vi "observacao_0MQ.vi"() -> ()   [LabVIEW 2012, in "Shared_160.lvlib"] (continued)
                n1514 = Multiply(x=0.01745329252 ("y"), y=w1906) -> (x*y=w1905:dbl)
                n1515 = Cosine(x=w1905) -> (cos(x)=w1894:dbl)
                n1516 = Sine(x=w1905) -> (sin(x)=w1895:dbl)
                n1517 = Multiply(x=w1892, y=w1894) -> (x*y=w1886:dbl)
                n1518 = Multiply(x=w1894, y=w1893) -> (x*y=w1891:dbl)
                n1519 = Multiply(x=w1893, y=w1895) -> (x*y=w1887:dbl)
                n1520 = Multiply(x=w1895, y=w1892) -> (x*y=w1890:dbl)
                n1521 = Subtract(x=w1891, y=w1890) -> (x-y=w1889:dbl)
                n1522 = Add(x=w1887, y=w1886) -> (x+y=w1888:dbl)
                n1523 = Less Than 0?(x=w1889) -> (x < 0?=w1903:bool)
                n1524 = Less Than 0?(x=w1888) -> (x < 0?=w1899:bool)
                n1525 = case shown="True" w1899 {
                  tunnel: w1897 -> [w1923 w1926]
                  tunnel: [w1922 w1927] -> w1896
                  frame False {
                    n1526 = Select(t="W" ("y"), s=w1923, f="E" ("y")) -> (s? t:f=w1922:string)
                  }
                  frame True {
                    n1527 = Select(t="E" ("y"), s=w1926, f="W" ("y")) -> (s? t:f=w1927:string)
                  }
                }
                n1528 = Select(t="S" ("y"), s=w1903, f="N" ("y")) -> (s? t:f=w1902:string)
                n1529 = Absolute Value(x=w1889) -> (abs(x)=w1900:dbl)
                n1530 = Absolute Value(x=w1888) -> (abs(x)=w1898:dbl)
                n1531 = global write "Global_Telescopio.vi" "guide_dir_we"(w1896) -> ()
                n1532 = global write "Global_Telescopio.vi" "guide_dir_ns"(w1902) -> ()
                n1533 = global write "Global_Telescopio.vi" "guide_dec"(w1900) -> ()
                n1534 = global write "Global_Telescopio.vi" "guide_asc"(w1898) -> ()
              }
            }
            "LED VAR TRACKING" <- "VARIABLE \nTRACKING"
          }
          frame "CALIBRATION" {
            # "Alterado dia 23/07/218"
            n1535 = disable-structure shown="Disabled" {
              frame Disabled {
              }
              frame Enabled {
              }
            }
            n1536 = disable-structure shown="Disabled" {
              frame Disabled {
                w1960 = u16 4 items=["ZERO", "AH", "DEC", "TUBO", "CUP"] ("Controlador")
                n1537 = call "Monta Comando.vi"("Comando"="FECHAR", "Dispositivo"="TRAPEIRA" ("Comando"), "Controlador"=w1960) -> ()  [unwired: 4 in, 3 out]
              }
              frame Enabled {
              }
            }
            n1538 = event shown="[4] \"Coude\": Value Change" {
              selector: _ -> [_ _ _ _ _]
              dyn-events: _ -> [_ _ _ _ _]
              timeout: 10 -> [_ _ _ _ _]
              event Timeout {
                n1539 = event-data() -> ()  [unwired: 1 in, 2 out]
              }
              event "Weak": Value Change {
                w1963 = u16 6 items=["Alarme", "Atencao", "Erro", "Ocupado", "TBD", "LCB", "Trapeira", "Paravento", "DomoRap", "DomoCW", "DomoCCW", "TBD", "Em movimento", "TBD"] ("NomeStatus")
                n1540 = event-data() -> ("NewVal"=w1964:bool)  [unwired: 1 in, 5 out]
                n1541 = call "Bit Status CUP.vi"("NomeStatus"=w1963) -> ("StatBit"=w1962:bool)
                n1542 = case shown="False" w1962 {
                  tunnel: w1964 -> [w1971 _]
                  frame False {
                    w1965 = u16 4 items=["ZERO", "AH", "DEC", "TUBO", "CUP"] ("Controlador")
                    n1543 = case shown="True" w1971 {
                      tunnel: [w1972 TRUE ("WeakSel")] -> w1970
                      tunnel: [w1972 FALSE ("MediumSel")] -> w1968
                      tunnel: [0 2] -> w1967
                      tunnel: ["DESLIGAR" ("Comando") "LIGAR" ("Comando")] -> w1969
                      frame False {
                        w1972 = FALSE ("MediumSel")
                      }
                      frame True {
                        n1544 = local write "DOME"(FALSE) -> ()
                        n1545 = local write "StatShutter"("Busy to Close" ("Status")) -> ()
                      }
                    }
                    n1546 = property on="Coude" class="Bool (strict)"("DisabledEnum"=w1967) -> ()  [unwired: 2 in, 2 out]
                    n1547 = property on="WeakSel" class="Bool (strict)"("Value"=w1970) -> ()  [unwired: 2 in, 2 out]
                    n1548 = property on="CoudeSel" class="Bool (strict)"("Value"=w1968) -> ()  [unwired: 2 in, 2 out]
                    n1549 = property on="Strong" class="Bool (strict)"("Disabled"=w1967) -> ()  [unwired: 2 in, 2 out]
                    n1550 = property on="MediumSel" class="Bool (strict)"("Value"=w1968) -> ()  [unwired: 2 in, 2 out]
                    n1551 = property on="StrongSel" class="Bool (strict)"("Value"=w1968) -> ()  [unwired: 2 in, 2 out]
                    n1552 = property on="Medium" class="Bool (strict)"("Disabled"=w1967) -> ()  [unwired: 2 in, 2 out]
                    n1553 = call "Monta Comando.vi"("Comando"=w1969, "Dispositivo"="FLAT_WEAK", "Controlador"=w1965) -> ()  [unwired: 4 in, 3 out]
                  }
                  frame True {
                    w1981 = FALSE ("Weak")
                    n1554 = Get Date/Time In Seconds() -> (seconds since 1Jan1904=w1984:timestamp)
                    n1555 = Add(x=w1984, y=10.0) -> (x+y=w1985:timestamp)
                    n1556 = property on="Weak" class="Bool (strict)"("Value"=w1981) -> ()  [unwired: 2 in, 2 out]
                    n1557 = local write "alarm Time"(w1985) -> ()
                    n1558 = property on="Mensage Alarme" class="Str"("Visible"=TRUE) -> ()  [unwired: 2 in, 2 out]
                    n1559 = property on="WeakSel" class="Bool (strict)"("Value"=w1981) -> ()  [unwired: 2 in, 2 out]
                    n1560 = local write "Flag Alarm"(TRUE ("Flag Alarm")) -> ()
                  }
                }
              }
              event "Medium": Value Change {
                w1988 = u16 6 items=["Alarme", "Atencao", "Erro", "Ocupado", "TBD", "LCB", "Trapeira", "Paravento", "DomoRap", "DomoCW", "DomoCCW", "TBD", "Em movimento", "TBD"] ("NomeStatus")
                n1561 = event-data() -> ("NewVal"=w1989:bool)  [unwired: 1 in, 5 out]
                n1562 = call "Bit Status CUP.vi"("NomeStatus"=w1988) -> ("StatBit"=w1987:bool)
                n1563 = case shown="False" w1987 {
                  tunnel: w1989 -> [w1996 _]
                  frame False {
                    w1991 = u16 4 items=["ZERO", "AH", "DEC", "TUBO", "CUP"] ("Controlador")
                    n1564 = case shown="True" w1996 {
                      tunnel: [0 2] -> w1993
                      tunnel: [w1998 TRUE] -> w1994
                      tunnel: [w1998 FALSE] -> w1992
                      tunnel: ["DESLIGAR" "LIGAR"] -> w1995
                      frame False {
                        w1998 = FALSE
                      }
                      frame True {
                        n1565 = local write "DOME"(FALSE) -> ()
                        n1566 = local write "StatShutter"("Busy to Close" ("Status")) -> ()
                      }
                    }
                    n1567 = property on="Weak" class="Bool (strict)"("Disabled"=w1993) -> ()  [unwired: 2 in, 2 out]
                    n1568 = property on="Strong" class="Bool (strict)"("Disabled"=w1993) -> ()  [unwired: 2 in, 2 out]
                    n1569 = property on="WeakSel" class="Bool (strict)"("Value"=w1992) -> ()  [unwired: 2 in, 2 out]
                    n1570 = property on="MediumSel" class="Bool (strict)"("Value"=w1994) -> ()  [unwired: 2 in, 2 out]
                    n1571 = property on="StrongSel" class="Bool (strict)"("Value"=w1992) -> ()  [unwired: 2 in, 2 out]
                    n1572 = property on="Coude" class="Bool (strict)"("DisabledEnum"=w1993) -> ()  [unwired: 2 in, 2 out]
                    n1573 = property on="CoudeSel" class="Bool (strict)"("Value"=w1992) -> ()  [unwired: 2 in, 2 out]
                    n1574 = call "Monta Comando.vi"("Comando"=w1995, "Dispositivo"="FLAT_LO", "Controlador"=w1991) -> ()  [unwired: 4 in, 3 out]
                  }
                  frame True {
                    w2006 = FALSE ("Medium")
                    n1575 = Get Date/Time In Seconds() -> (seconds since 1Jan1904=w2009:timestamp)
                    n1576 = Add(x=w2009, y=10.0) -> (x+y=w2010:timestamp)
                    n1577 = local write "alarm Time"(w2010) -> ()
                    n1578 = property on="Mensage Alarme" class="Str"("Visible"=TRUE) -> ()  [unwired: 2 in, 2 out]
                    n1579 = local write "Flag Alarm"(TRUE ("Flag Alarm")) -> ()
                    n1580 = property on="Medium" class="Bool (strict)"("Value"=w2006) -> ()  [unwired: 2 in, 2 out]
                    n1581 = property on="MediumSel" class="Bool (strict)"("Value"=w2006) -> ()  [unwired: 2 in, 2 out]
                  }
                }
              }
              event "Strong": Value Change {
                w2013 = u16 6 items=["Alarme", "Atencao", "Erro", "Ocupado", "TBD", "LCB", "Trapeira", "Paravento", "DomoRap", "DomoCW", "DomoCCW", "TBD", "Em movimento", "TBD"] ("NomeStatus")
                n1582 = event-data() -> ("NewVal"=w2014:bool)  [unwired: 1 in, 5 out]
                n1583 = call "Bit Status CUP.vi"("NomeStatus"=w2013) -> ("StatBit"=w2012:bool)
                n1584 = case shown="False" w2012 {
                  tunnel: w2014 -> [w2022 _]
                  frame False {
                    w2015 = u16 4 items=["ZERO", "AH", "DEC", "TUBO", "CUP"] ("Controlador")
                    n1585 = case shown="True" w2022 {
                      tunnel: [FALSE w2030] -> w2017
                      tunnel: [w2023 w2030] -> w2021
                      tunnel: [0 2] -> w2018
                      tunnel: ["DESLIGAR" "LIGAR"] -> w2020
                      tunnel: [w2023 TRUE] -> w2019
                      frame False {
                        w2023 = FALSE
                      }
                      frame True {
                        w2030 = FALSE
                        n1586 = local write "DOME"(FALSE) -> ()
                        n1587 = local write "StatShutter"("Busy to Close" ("Status")) -> ()
                      }
                    }
                    n1588 = property on="Medium" class="Bool (strict)"("Disabled"=w2018) -> ()  [unwired: 2 in, 2 out]
                    n1589 = property on="Weak" class="Bool (strict)"("Disabled"=w2018) -> ()  [unwired: 2 in, 2 out]
                    n1590 = property on="WeakSel" class="Bool (strict)"("Value"=w2021) -> ()  [unwired: 2 in, 2 out]
                    n1591 = property on="MediumSel" class="Bool (strict)"("Value"=w2017) -> ()  [unwired: 2 in, 2 out]
                    n1592 = property on="StrongSel" class="Bool (strict)"("Value"=w2019) -> ()  [unwired: 2 in, 2 out]
                    n1593 = property on="Coude" class="Bool (strict)"("DisabledEnum"=w2018) -> ()  [unwired: 2 in, 2 out]
                    n1594 = property on="CoudeSel" class="Bool (strict)"("Value"=w2017) -> ()  [unwired: 2 in, 2 out]
                    n1595 = call "Monta Comando.vi"("Comando"=w2020, "Dispositivo"="FLAT_HI", "Controlador"=w2015) -> ()  [unwired: 4 in, 3 out]
                  }
                  frame True {
                    w2033 = FALSE ("Strong")
                    n1596 = property on="StrongSel" class="Bool (strict)"("Value"=w2033) -> ()  [unwired: 2 in, 2 out]
                    n1597 = property on="Strong" class="Bool (strict)"("Value"=w2033) -> ()  [unwired: 2 in, 2 out]
                    n1598 = Get Date/Time In Seconds() -> (seconds since 1Jan1904=w2036:timestamp)
                    n1599 = Add(x=w2036, y=10.0) -> (x+y=w2037:timestamp)
                    n1600 = local write "alarm Time"(w2037) -> ()
                    n1601 = property on="Mensage Alarme" class="Str"("Visible"=TRUE) -> ()  [unwired: 2 in, 2 out]
                    n1602 = local write "Flag Alarm"(TRUE ("Flag Alarm")) -> ()
                  }
                }
              }
              event "Coude": Value Change {
                w2040 = u16 6 items=["Alarme", "Atencao", "Erro", "Ocupado", "TBD", "LCB", "Trapeira", "Paravento", "DomoRap", "DomoCW", "DomoCCW", "TBD", "Em movimento", "TBD"] ("NomeStatus")
                n1603 = event-data() -> ("NewVal"=w2041:bool)  [unwired: 1 in, 5 out]
                n1604 = call "Bit Status CUP.vi"("NomeStatus"=w2040) -> ("StatBit"=w2039:bool)
                n1605 = case shown="False" w2039 {
                  tunnel: w2041 -> [w2048 _]
                  frame False {
                    w2042 = u16 4 items=["ZERO", "AH", "DEC", "TUBO", "CUP"] ("Controlador")
                    n1606 = case shown="True" w2048 {
                      tunnel: [FALSE w2057] -> w2045
                      tunnel: [w2050 w2057] -> w2046
                      tunnel: [0 2] -> w2044
                      tunnel: ["DESLIGAR" "LIGAR"] -> w2049
                      tunnel: [w2050 TRUE] -> w2047
                      frame False {
                        w2050 = FALSE
                      }
                      frame True {
                        w2057 = FALSE
                        n1607 = local write "DOME"(FALSE) -> ()
                        n1608 = local write "StatShutter"("Busy to Close" ("Status")) -> ()
                      }
                    }
                    n1609 = property on="StrongSel" class="Bool (strict)"("Value"=w2046) -> ()  [unwired: 2 in, 2 out]
                    n1610 = property on="CoudeSel" class="Bool (strict)"("Value"=w2047) -> ()  [unwired: 2 in, 2 out]
                    n1611 = property on="MediumSel" class="Bool (strict)"("Value"=w2045) -> ()  [unwired: 2 in, 2 out]
                    n1612 = property on="Weak" class="Bool (strict)"("DisabledEnum"=w2044) -> ()  [unwired: 2 in, 2 out]
                    n1613 = property on="Medium" class="Bool (strict)"("DisabledEnum"=w2044) -> ()  [unwired: 2 in, 2 out]
                    n1614 = property on="Strong" class="Bool (strict)"("DisabledEnum"=w2044) -> ()  [unwired: 2 in, 2 out]
                    n1615 = property on="WeakSel" class="Bool (strict)"("Value"=w2045) -> ()  [unwired: 2 in, 2 out]
                    n1616 = call "Monta Comando.vi"("Comando"=w2049, "Dispositivo"="FLAT_COUDE", "Controlador"=w2042) -> ()  [unwired: 4 in, 3 out]
                  }
                  frame True {
                    w2060 = FALSE ("Coude")
                    n1617 = Get Date/Time In Seconds() -> (seconds since 1Jan1904=w2063:timestamp)
                    n1618 = Add(x=w2063, y=10.0) -> (x+y=w2064:timestamp)
                    n1619 = local write "alarm Time"(w2064) -> ()
                    n1620 = property on="Mensage Alarme" class="Str"("Visible"=TRUE) -> ()  [unwired: 2 in, 2 out]
                    n1621 = local write "Flag Alarm"(TRUE ("Flag Alarm")) -> ()
                    n1622 = property on="CoudeSel" class="Bool (strict)"("Value"=w2060) -> ()  [unwired: 2 in, 2 out]
                    n1623 = property on="Coude" class="Bool (strict)"("Value"=w2060) -> ()  [unwired: 2 in, 2 out]
                  }
                }
              }
            }
          }
          frame "LIST" {
            n1624 = stacked-sequence {
              frame #0 {
                # "Muda nome do controle de RA para AH se MAFmax == 100"
                n1625 = case shown="True" "SET coord" {
                  frame False {
                  }
                  frame True {
                    n1626 = stacked-sequence {
                      frame #0 {
                        w2081 = "2000"
                        # "Valores aux para Detectar Edição"
                        n1627 = local read "Multicolumn Listbox"() -> (w2088:i32[])
                        n1628 = property on="Multicolumn Listbox" class="MCListbox (strict)"() -> ("Item Names"=w2086:string[][])  [unwired: 2 in, 2 out]
                        n1629 = Index Array(array=w2088, index=0) -> (element=w2085:i32)
                        n1630 = local write "FLAG SET COORD"(TRUE ("FLAG_MAG")) -> ()
                        n1631 = Index Array(array=w2086, index (row)=w2085) -> (element=w2084:string[])  [unwired: 1 in]
                        n1632 = Index Array(array=w2084, index #1=0 ("index")) -> (element #1=w2077:string, element #2=w2075:string, element #3=w2076:string, element #4=w2078:string, element #5=w2080:string, element #6=w2079:string)  [unwired: 5 in]
                        "RA AUX" <- w2075
                        "AUX EDITA Name" <- w2077
                        "AUX EDITA RA" <- w2075
                        "AUX EDITA DEC" <- w2076
                        "AUX EDITA PMRA" <- w2080
                        "AUX EDITA PMDEC" <- w2079
                        n1633 = local write "StrPointObjPMRA"(w2080) -> ()
                        n1634 = local write "StrPointObjPMDEC"(w2079) -> ()
                        n1635 = local write "StrPointObjName"(w2077) -> ()
                        n1636 = local write "StrPointObjRA"(w2075) -> ()
                        n1637 = local write "StrPointObjDEC"(w2076) -> ()
                        n1638 = local write "MAG"(w2078) -> ()
                        n1639 = local write "StrPointObjEpoch"(w2081) -> ()
                        "EPOCH AUX" <- w2081
                        "AUX EDITA EPOCH" <- w2081
                      }
                      frame #1 {
                        n1640 = case shown="False" "Case Constant\n(See Context Help) 7" {
                          frame False {
                          }
                          frame True {
                            # "Ao clicar SET COORD, fechar a aba LIST e abrir a aba POINTING"
                            n1641 = local write "Setup, Pointing & Guiding"(T2."POINTING" ("Setup, Pointing & Guiding")) -> ()
                          }
                        }
                      }
                    }
                  }
                }
                n1642 = case shown="True" "Clear ALL" {
                  frame False {
                  }
                  frame True {
                    n1643 = Two Button Dialog(message="Will you clear All Table?") -> (T button?=w2091:bool)  [unwired: 2 in]
                    n1644 = case shown="True" w2091 {
                      frame False {
                      }
                      frame True {
                        w2093 = string[][] [] ("Item Names")
                        # "Limpa a Tabela Inteira"
                        n1645 = property on="Multicolumn Listbox" class="MCListbox (strict)"("Item Names"=w2093) -> ()  [unwired: 2 in, 2 out]
                        n1646 = local write "subarray"(w2093) -> ()
                      }
                    }
                  }
                }
                n1647 = local read "MAG Max"() -> (w2067:dbl)
                n1648 = Equal?(x=100.0, y=w2067) -> (x = y?=w2066:bool)
                n1649 = case shown="False" w2066 {
                  frame False {
                    n1650 = flat-sequence {
                      frame #0 {
                        w2071 = FALSE
                        n1651 = property on="RA Max" class="DigNum (strict)"("Caption.Visible"=w2071) -> ()  [unwired: 2 in, 2 out]
                        n1652 = property on="RA Min" class="DigNum (strict)"("Caption.Visible"=w2071) -> ()  [unwired: 2 in, 2 out]
                      }
                      frame #1 {
                        w2072 = TRUE
                        n1653 = property on="RA Min" class="DigNum (strict)"("Label.Visible"=w2072) -> ()  [unwired: 2 in, 2 out]
                        n1654 = property on="RA Max" class="DigNum (strict)"("Label.Visible"=w2072) -> ()  [unwired: 2 in, 2 out]
                      }
                    }
                  }
                  frame True {
                    n1655 = flat-sequence {
                      frame #0 {
                        w2073 = FALSE
                        n1656 = property on="RA Max" class="DigNum (strict)"("Label.Visible"=w2073) -> ()  [unwired: 2 in, 2 out]
                        n1657 = property on="RA Min" class="DigNum (strict)"("Label.Visible"=w2073) -> ()  [unwired: 2 in, 2 out]
                      }
                      frame #1 {
                        w2074 = TRUE
                        n1658 = property on="RA Min" class="DigNum (strict)"("Caption.Visible"=w2074) -> ()  [unwired: 2 in, 2 out]
                        n1659 = property on="RA Max" class="DigNum (strict)"("Caption.Visible"=w2074) -> ()  [unwired: 2 in, 2 out]
                      }
                    }
                  }
                }
              }
              frame #1 {
                # "MUDANÇA:\nUPLOAD carrega\ncatálogo usuário"
                n1660 = case shown="True" "Upload" {
                  frame False {
                  }
                  frame True {
                    n1661 = File Dialog() -> (0:w2099:errorcluster, 1:w2101:bool, 3:w2100:path)  [unwired: 7 in, 1 out]
                    n1662 = Unbundle(w2099) -> ("status"=w2098:bool)  [unwired: 2 out]
                    n1663 = Not(x=w2098) -> (.not. x?=w2096:bool)
                    n1664 = And(x=w2101, y=w2096) -> (x .and. y?=w2097:bool)
                    n1665 = case shown="False" w2097 {
                      tunnel: w2100 -> [w2105 _]
                      frame False {
                        w2106 = 0 ("Slide")
                        # "Abre Arquivo Escolhido"
                        n1666 = Strip Path(path=w2105) -> (name=w2103:string)  [unwired: 1 out]
                        n1667 = Path To String(path=w2105) -> (string=w2109:string)
                        n1668 = local write "List File"(w2103) -> ()
                        n1669 = call "leexel.vi"("path"=w2109) -> ("array 5"=w2104:string[][])  [unwired: 4 in]
                        n1670 = local write "Slide"(w2106) -> ()
                        n1671 = local write "subarray"(w2104) -> ()
                        n1672 = Array Subset(array=w2104, index (row)=w2106, length (row)=10 ("length"), index (col)=w2106, length (col)=8 ("index")) -> (w2102:string[][])
                        n1673 = property on="Multicolumn Listbox" class="MCListbox (strict)"("Item Names"=w2102) -> ()  [unwired: 2 in, 2 out]
                      }
                      frame True {
                      }
                    }
                  }
                }
                n1674 = case shown="True" "Save AS" {
                  frame False {
                  }
                  frame True {
                    n1675 = File Dialog() -> (0:w2110:errorcluster, 1:w2112:bool, 3:w2111:path)  [unwired: 7 in, 1 out]
                    n1676 = Unbundle(w2110) -> ()  [unwired: 3 out]
                    n1677 = case shown="False" w2112 {
                      tunnel: w2111 -> [w2114 _]
                      frame False {
                        # "Salva Arquivo Escolhido"
                        n1678 = Path To String(path=w2114) -> (string=w2115:string)
                        n1679 = case shown="True" "Case Constant\n(See Context Help) 8" {
                          tunnel: w2115 -> [_ w2117]
                          frame False {
                          }
                          frame True {
                            n1680 = local read "subarray"() -> (w2116:string[][])
                            n1681 = call "salvaexel.vi"("appended array"=w2116, "file name p/ exell"=w2117) -> ()  [unwired: 1 in, 1 out]
                          }
                        }
                      }
                      frame True {
                      }
                    }
                  }
                }
              }
              frame #2 {
                # "Acerta Posição do Slide"
                n1682 = local read "Tot Linhas"() -> (w2123:i32)
                n1683 = Multiply(x="Slide", y=w2123) -> (x*y=w2122:dbl)
                n1684 = Divide(x=w2122, y=24.0) -> (x/y=w2120:dbl)
                n1685 = Not Equal?(x=w2120, y="Slide old") -> (x != y?=w2125:bool)
                n1686 = case shown="True" w2125 {
                  tunnel: w2120 -> [_ w2130]
                  frame False {
                  }
                  frame True {
                    n1687 = stacked-sequence {
                      seq-local: [w2134 _] -> [_ w2139]
                      tunnel: w2130 -> [w2135 _]
                      frame #0 {
                        # "Previne estouro\nda planilha"
                        n1688 = local read "Tot Linhas"() -> (w2133:i32)
                        n1689 = Subtract(x=w2133, y=10) -> (x-y=w2131:i32)
                        n1690 = Greater Or Equal?(x=w2135, y=w2131) -> (x >= y?=w2136:bool)
                        n1691 = case shown="False" w2136 {
                          tunnel: [w2137 w2138] -> w2134
                          tunnel: w2131 -> [_ w2138]
                          tunnel: w2135 -> [w2137 _]
                          frame False {
                          }
                          frame True {
                          }
                        }
                      }
                      frame #1 {
                        n1692 = local read "subarray"() -> (w2141:string[][])
                        n1693 = Array Subset(array=w2141, index (row)=w2139, length (row)=11 ("length"), index (col)=0 ("index"), length (col)=8 ("index")) -> (w2140:string[][])
                        n1694 = property on="Multicolumn Listbox" class="MCListbox (strict)"("Item Names"=w2140) -> ()  [unwired: 2 in, 2 out]
                        n1695 = local write "Slide old"(w2139) -> ()
                      }
                    }
                  }
                }
                n1696 = case shown="True" "Open BSC" {
                  frame False {
                  }
                  frame True {
                    n1697 = stacked-sequence {
                      frame #0 {
                        w2178 = FALSE
                        # "MUDANÇA:\nUPLOAD carrega\ncatálogo usuário"
                        # "Faz Aparecer os Botões"
                        n1698 = property on="Delete" class="Bool"("Visible"=w2178) -> ()  [unwired: 2 in, 2 out]
                        n1699 = property on="EDIT" class="Bool"("Visible"=w2178) -> ()  [unwired: 2 in, 2 out]
                        n1700 = property on="Clear ALL" class="Bool"("Visible"=w2178) -> ()  [unwired: 2 in, 2 out]
                        n1701 = property on="Save AS" class="Bool"("Visible"=w2178) -> ()  [unwired: 2 in, 2 out]
                        n1702 = property on="Save" class="Bool"("Visible"=w2178) -> ()  [unwired: 2 in, 2 out]
                        n1703 = property on="Insert" class="Bool"("Visible"=w2178) -> ()  [unwired: 2 in, 2 out]
                        n1704 = property on="Upload" class="Bool"("Visible"=TRUE) -> ()  [unwired: 2 in, 2 out]
                      }
                      frame #1 {
                        w2179 = "C:\\TCS\\ARQUIVOS\\BSC_08.txt"
                        w2186 = 0 ("Slide")
                        # "Cria e Lê arquivo\nonde voce está\ntrabalhando"
                        n1705 = local write "Slide"(w2186) -> ()
                        n1706 = call "leexel.vi"("path"=w2179) -> ("array 5"=w2184:string[][])  [unwired: 4 in]
                        "subarray" <- w2184
                        n1707 = Array Subset(array=w2184, index (row)=w2186, length (row)=11 ("length"), index (col)=w2186, length (col)=8 ("index")) -> (w2187:string[][])
                        n1708 = Array Size(array=w2184) -> (size(s)=w2185:i32[])
                        n1709 = String To Path(string=w2179) -> (path=w2181:path)
                        n1710 = property on="Multicolumn Listbox" class="MCListbox (strict)"("Item Names"=w2187) -> ()  [unwired: 2 in, 2 out]
                        n1711 = Strip Path(path=w2181) -> (name=→"List File":string)  [unwired: 1 out]
                        n1712 = Index Array(array=w2185, index=0) -> (element=→"Tot Linhas":i32)
                        "Saida Path string" <- w2179
                      }
                      frame #2 {
                        n1713 = local read "Tot Linhas"() -> (w2198:i32)
                        n1714 = Quotient & Remainder(x=10000, y=w2198) -> (floor(x/y)=w2196:i32)  [unwired: 1 out]
                        n1715 = Divide(x=w2196, y=1000) -> (x/y=w2193:dbl)
                        n1716 = Multiply(x=w2193, y=24.0) -> (x*y=w2194:dbl)
                        n1717 = property on="Slide" class="Slide (strict)"("Data Entry Limits:Increment"=w2194) -> ()  [unwired: 2 in, 2 out]
                        "ScaleMax" <- "24" ("ScaleMax")
                        "ScaleMin" <- "0" ("ScaleMin")
                      }
                    }
                  }
                }
                n1718 = case shown="True" "Save" {
                  frame False {
                  }
                  frame True {
                    w2173 = "C:\\TCS\\ARQUIVOS\\List.lst"
                    # "Cria e Lê arquivo\nonde voce está\ntrabalhando"
                    n1719 = String To Path(string=w2173) -> (path=w2172:path)
                    n1720 = stacked-sequence {
                      tunnel: w2172 -> [w2174 _]
                      tunnel: w2173 -> [_ w2176]
                      frame #0 {
                        # "Apaga o arquivo"
                        n1721 = Delete(path (use dialog)=w2174) -> ()  [unwired: 4 in, 3 out]
                      }
                      frame #1 {
                        # "Salva a lista"
                        n1722 = local read "subarray"() -> (w2175:string[][])
                        n1723 = call "salvaexel.vi"("appended array"=w2175, "file name p/ exell"=w2176) -> ()  [unwired: 1 in, 1 out]
                      }
                    }
                  }
                }
                n1724 = case shown="True" "Delete" {
                  frame False {
                  }
                  frame True {
                    n1725 = local read "Multicolumn Listbox"() -> (w2151:i32[])
                    n1726 = Index Array(array=w2151, index=0) -> (element=w2145:i32)
                    n1727 = Number To Decimal String(number=w2145) -> (decimal integer string=w2148:string)  [unwired: 1 in]
                    n1728 = Concatenate Strings("Delete Line Number: " ("string"), w2148) -> (w2146:string)
                    n1729 = Two Button Dialog(message=w2146) -> (T button?=w2147:bool)  [unwired: 2 in]
                    n1730 = case shown="True" w2147 {
                      tunnel: w2145 -> [_ w2152]
                      frame False {
                      }
                      frame True {
                        n1731 = stacked-sequence {
                          tunnel: w2152 -> [w2156 _]
                          frame #0 {
                            # "Apaga a Coluna Escolhida"
                            n1732 = property on="Multicolumn Listbox" class="MCListbox (strict)"() -> ("Item Names"=w2159:string[][])  [unwired: 2 in, 2 out]
                            n1733 = local read "Slide"() -> (w2157:dbl)
                            n1734 = local read "subarray"() -> (w2154:string[][])
                            n1735 = Add(x=w2156, y=w2157) -> (x+y=w2155:dbl)
                            n1736 = Delete From Array(array=w2159, index (row)=w2156) -> (array with subset deleted=w2158:string[][])  [unwired: 2 in, 1 out]
                            n1737 = Delete From Array(array=w2154, index (row)=w2155) -> (array with subset deleted=w2153:string[][])  [unwired: 2 in, 1 out]
                            n1738 = local write "subarray"(w2153) -> ()
                            n1739 = property on="Multicolumn Listbox" class="MCListbox (strict)"("Item Names"=w2158) -> ()  [unwired: 2 in, 2 out]
                          }
                          frame #1 {
                            # "Volta para a coluna Zero"
                            n1740 = local write "Multicolumn Listbox"(i32[] [0] ("Multicolumn Listbox")) -> ()
                          }
                        }
                      }
                    }
                  }
                }
                n1741 = case shown="True" "Insert" {
                  frame False {
                  }
                  frame True {
                    n1742 = stacked-sequence {
                      seq-local: [w2162 _ _] -> [_ w2164 _]
                      seq-local: [w2161 _ _] -> [_ w2163 _]
                      frame #0 {
                        n1743 = call "Tela_Set_Coordenadas.vi"() -> ("Saída"=w2162:bool, "Val Saída"=w2161:string[])  [unwired: 4 in]
                      }
                      frame #1 {
                        n1744 = case shown="True" w2164 {
                          tunnel: w2163 -> [_ w2165]
                          frame False {
                          }
                          frame True {
                            # "Insere Linha Preenchida"
                            n1745 = local read "subarray"() -> (w2167:string[][])
                            n1746 = property on="Multicolumn Listbox" class="MCListbox (strict)"() -> ("Item Names"=w2169:string[][])  [unwired: 2 in, 2 out]
                            n1747 = Build Array (concatenate)(w2169, w2165) -> (w2168:string[][])
                            n1748 = Build Array (concatenate)(w2167, w2165) -> (w2166:string[][])
                            n1749 = property on="Multicolumn Listbox" class="MCListbox (strict)"("Item Names"=w2168) -> ()  [unwired: 2 in, 2 out]
                            n1750 = local write "subarray"(w2166) -> ()
                          }
                        }
                      }
                      frame #2 {
                        # "Depois de inserir um novo objeto na tabela,\n com o comando INSERT, mudar o objeto \nselecionado para esse novo registro."
                        n1751 = property on="Multicolumn Listbox" class="MCListbox (strict)"() -> ("Number of Rows"=w2171:u32)  [unwired: 2 in, 2 out]
                        n1752 = Build Array(w2171) -> (w2170:u32[])
                        n1753 = local write "Multicolumn Listbox"(w2170) -> ()
                      }
                    }
                  }
                }
                n1754 = property on="Multicolumn Listbox" class="MCListbox (strict)"("Selection Color"=u32 10336195) -> ()  [unwired: 2 in, 2 out]
              }
              frame #3 {
                # "Editar a Lista"
                n1755 = case shown="True" "EDIT" {
                  frame False {
                  }
                  frame True {
                    (unwired) "Edit the marked Line and soon after presses SAVE"
                    n1756 = call "Edita_lista.vi"() -> ("lista Auxiliar"=w2221:string[][])  [unwired: 5 in]
                    n1757 = property on="Multicolumn Listbox" class="MCListbox (strict)"("Item Names"=w2221) -> ()  [unwired: 2 in, 2 out]
                  }
                }
                n1758 = case shown="True" "Open" {
                  frame False {
                  }
                  frame True {
                    n1759 = stacked-sequence {
                      frame #0 {
                        w2201 = TRUE
                        # "Faz Aparecer os Botões"
                        n1760 = property on="Delete" class="Bool"("Visible"=w2201) -> ()  [unwired: 2 in, 2 out]
                        n1761 = property on="EDIT" class="Bool"("Visible"=w2201) -> ()  [unwired: 2 in, 2 out]
                        n1762 = property on="Clear ALL" class="Bool"("Visible"=w2201) -> ()  [unwired: 2 in, 2 out]
                        n1763 = property on="Upload" class="Bool"("Visible"=w2201) -> ()  [unwired: 2 in, 2 out]
                        n1764 = property on="Save AS" class="Bool"("Visible"=w2201) -> ()  [unwired: 2 in, 2 out]
                        n1765 = property on="Save" class="Bool"("Visible"=w2201) -> ()  [unwired: 2 in, 2 out]
                        n1766 = property on="Insert" class="Bool"("Visible"=w2201) -> ()  [unwired: 2 in, 2 out]
                      }
                      frame #1 {
                        w2209 = 0 ("Slide")
                        w2205 = "C:\\TCS\\ARQUIVOS\\List.lst"
                        n1767 = String To Path(string=w2205) -> (path=w2212:path)
                        n1768 = local write "Saida Path string"(w2205) -> ()
                        n1769 = call "leexel.vi"("path"=w2205) -> ("array 5"=w2204:string[][])  [unwired: 4 in]
                        n1770 = Strip Path(path=w2212) -> (name=w2211:string)  [unwired: 1 out]
                        n1771 = local write "List File"(w2211) -> ()
                        n1772 = local write "subarray"(w2204) -> ()
                        n1773 = Array Subset(array=w2204, index (row)=w2209, length (row)=10 ("length"), index (col)=w2209, length (col)=8 ("index")) -> (w2208:string[][])
                        n1774 = local write "Slide"(w2209) -> ()
                        n1775 = Array Size(array=w2204) -> (size(s)=w2202:i32[])
                        n1776 = property on="Multicolumn Listbox" class="MCListbox (strict)"("Item Names"=w2208) -> ()  [unwired: 2 in, 2 out]
                        n1777 = Index Array(array=w2202, index=0) -> (element=w2203:i32)
                        n1778 = local write "Tot Linhas"(w2203) -> ()
                      }
                      frame #2 {
                        w2213 = ""
                        n1779 = local read "Tot Linhas"() -> (w2220:i32)
                        n1780 = Quotient & Remainder(x=10000, y=w2220) -> (floor(x/y)=w2218:i32)  [unwired: 1 out]
                        n1781 = Divide(x=w2218, y=1000) -> (x/y=w2215:dbl)
                        n1782 = Multiply(x=w2215, y=24.0) -> (x*y=w2216:dbl)
                        n1783 = property on="Slide" class="Slide (strict)"("Data Entry Limits:Increment"=w2216) -> ()  [unwired: 2 in, 2 out]
                        n1784 = local write "ScaleMin"(w2213) -> ()
                        n1785 = local write "ScaleMax"(w2213) -> ()
                      }
                    }
                  }
                }
              }
              frame #4 {
                n1786 = case shown="True" "Filter RA" {
                  frame False {
                  }
                  frame True {
                    n1787 = while {
                      shift-right: [w2224] -> _
                      shift-left: "inicio" -> [w2226]
                      stop <- w2225 stop-if-true
                      n1788 = case shown="\"filtra\"" w2226 {
                        tunnel: [FALSE w2276 TRUE TRUE] -> w2225
                        tunnel: [w2246 w2277 "fim" "fim"] -> w2224
                        frame "inicio" {
                          # "RAmin"
                          # "RAmax"
                          # "Testa se:\n| Ramax - Ramin | >=1\n|Decmax -Decmin | >=1\n|Magmax -Magmin | >=1"
                          n1789 = local read "MAG Max"() -> (w2240:dbl)
                          n1790 = local read "MAG Min"() -> (w2255:dbl)
                          n1791 = Equal?(x=100.0, y=w2240) -> (x = y?=w2232:bool)
                          n1792 = Subtract(x=w2240, y=w2255) -> (x-y=w2252:dbl)
                          n1793 = case shown="True" w2232 {
                            tunnel: "RA Min" -> [w2260 w2268]
                            tunnel: [w2260 w2267] -> w2227
                            tunnel: "RA Max" -> [w2259 w2269]
                            tunnel: [w2259 w2264] -> w2228
                            frame False {
                            }
                            frame True {
                              w2273 = 24 ("RA Max")
                              # "12h/PI()"
                              # "TS, rad"
                              # "TS, hora"
                              # "RAmin"
                              # "RAmax"
                              # "AHmax"
                              # "AHmin"
                              # "MUDANÇA 7/4/2011:\nSe MAGmax >= 100,\ntratar RA como AH."
                              n1794 = global read "Global_Telescopio.vi" "Sideral Time"() -> (w2263:dbl)
                              n1795 = Multiply(x=w2263, y=3.8197) -> (x*y=w2262:dbl)
                              n1796 = To Long Integer(number=w2262) -> (32bit integer=w2270:i32)
                              n1797 = Subtract(x=w2270, y=w2269) -> (x-y=w2266:i32)
                              n1798 = Subtract(x=w2270, y=w2268) -> (x-y=w2265:i32)
                              n1799 = Add(x=w2273, y=w2266) -> (x+y=w2272:i32)
                              n1800 = Less Than 0?(x=w2266) -> (x < 0?=w2275:bool)
                              n1801 = Add(x=w2273, y=w2265) -> (x+y=w2271:i32)
                              n1802 = Less Than 0?(x=w2265) -> (x < 0?=w2274:bool)
                              n1803 = Select(t=w2272, s=w2275, f=w2266) -> (s? t:f=w2267:i32)
                              n1804 = Select(t=w2271, s=w2274, f=w2265) -> (s? t:f=w2264:i32)
                            }
                          }
                          n1805 = Less?(x=w2252, y=1.0) -> (x < y?=w2249:bool)
                          n1806 = local read "DEC Max"() -> (w2257:i32)
                          n1807 = local read "DEC Min"() -> (w2256:i32)
                          n1808 = local write "RA Min 2"(w2227) -> ()
                          n1809 = local write "RA Max 2"(w2228) -> ()
                          n1810 = Less?(x=w2228, y=w2227) -> (x < y?=w2233:bool)
                          "FiltroDuplo" <- w2233
                          n1811 = Equal?(x=w2228, y=w2227) -> (x = y?=w2231:bool)
                          n1812 = Add(x=w2228, y=24 ("RA Max")) -> (x+y=w2237:i32)
                          n1813 = Subtract(x=w2237, y=w2227) -> (x-y=w2236:i32)
                          n1814 = Subtract(x=w2257, y=w2256) -> (x-y=w2254:i32)
                          n1815 = Greater?(x=w2236, y=12) -> (0:w2234:bool)
                          n1816 = control-ref of="Erro"() -> (w2243:refnum<vi>)
                          n1817 = Less?(x=w2254, y=1) -> (x < y?=w2250:bool)
                          n1818 = And(x=w2234, y=w2233) -> (x .and. y?=w2241:bool)
                          n1819 = property class="Bool (strict)"(reference=w2243, "Boolean Text.Text"="WAIT") -> ()  [unwired: 1 in, 2 out]
                          n1820 = Compound Arithmetic op=OR(w2241, w2231, w2250, w2249) -> (w2248:bool)
                          n1821 = Select(t="erro", s=w2248, f="filtra") -> (s? t:f=w2246:string)
                          "Erro" <- FALSE ("Fim")
                        }
                        frame "filtra" {
                          n1822 = stacked-sequence {
                            seq-local: [w2281 _ _ _] -> [_ w2324 _ _]
                            seq-local: [_ w2325 _ _] -> [_ _ w2344 _]
                            seq-local: [_ _ w2345 _] -> [_ _ _ w2370]
                            tunnel: [_ _ _ "fim"] -> w2277
                            tunnel: [_ _ _ FALSE] -> w2276
                            frame #0 {
                              n1823 = property on="EDIT" class="Bool"() -> ("Visible"=w2278:bool)  [unwired: 2 in, 2 out]
                              n1824 = case shown="True" w2278 {
                                tunnel: ["C:\\TCS\\ARQUIVOS\\BSC_08.txt" "C:\\TCS\\ARQUIVOS\\List.lst"] -> w2280
                                frame False {
                                }
                                frame True {
                                }
                              }
                              n1825 = call "leexel.vi"("path"=w2280) -> ("array 5"=w2279:string[][])  [unwired: 4 in]
                              n1826 = Index Array(array=w2279, index (col)=1 ("disabled index (col)")) -> (element=w2283:string[])  [unwired: 1 in]
                              n1827 = for {
                                tunnel: w2283 -> [w2299] mode=indexing
                                shift-right: [w2293] -> w2281
                                shift-left: string[][] [] ("Item Names") -> [w2295]
                                tunnel: w2279 -> [w2292] mode=indexing
                                # "Filtro de RA"
                                n1828 = local read "FiltroDuplo"() -> (w2291:bool)
                                n1829 = String Subset(string=w2299, offset (0)=0, length (rest)=2 ("length (rest)")) -> (substring=w2296:string)
                                n1830 = Decimal String To Number(string=w2296) -> (number=w2290:i32)  [unwired: 2 in, 1 out]
                                n1831 = case shown="False" w2291 {
                                tunnel: "RA Max 2" -> [w2304 w2309]
                                tunnel: "RA Min 2" -> [w2303 w2306]
                                tunnel: [w2302 w2311] -> w2294
                                tunnel: w2290 -> [w2301 w2310]
                                tunnel: [FALSE w2305] -> w2289
                                frame False {
                                n1832 = In Range and Coerce(upper limit=w2304, x=w2301, lower limit=w2303) -> (In Range?=w2302:bool)  [unwired: 1 out]
                                }
                                frame True {
                                n1833 = In Range and Coerce(upper limit=w2309, x=w2310, lower limit=0 ("upper limit")) -> (In Range?=w2312:bool)  [unwired: 1 out]
                                n1834 = In Range and Coerce(upper limit=24 ("lower limit"), x=w2310, lower limit=w2306) -> (In Range?=w2305:bool)  [unwired: 1 out]
                                n1835 = Or(x=w2312, y=w2305) -> (x .or. y?=w2311:bool)
                                }
                                }
                                n1836 = case shown="True" w2294 {
                                tunnel: w2295 -> [w2313 w2317]
                                tunnel: [w2313 w2316] -> w2293
                                tunnel: w2292 -> [_ w2315]
                                tunnel: w2289 -> [_ w2314]
                                frame False {
                                }
                                frame True {
                                n1837 = case shown="False" w2314 {
                                tunnel: w2317 -> [w2320 w2322]
                                tunnel: [w2319 w2321] -> w2316
                                tunnel: w2315 -> [w2318 w2323]
                                frame False {
                                n1838 = Build Array (concatenate)(w2320, w2318) -> (w2319:string[][])
                                }
                                frame True {
                                n1839 = Build Array (concatenate)(w2323, w2322) -> (w2321:string[][])
                                }
                                }
                                }
                                }
                              }
                            }
                            frame #1 {
                              # "Filtro de DEC"
                              n1840 = Index Array(array=w2324, index (col)=2 ("disabled index (col)")) -> (element=w2327:string[])  [unwired: 1 in]
                              n1841 = for {
                                tunnel: w2327 -> [w2339] mode=indexing
                                shift-right: [w2332] -> w2325
                                shift-left: string[][] [] ("Item Names") -> [w2334]
                                tunnel: w2324 -> [w2331] mode=indexing
                                n1842 = String Subset(string=w2339, offset (0)=0, length (rest)=3 ("length (rest)")) -> (substring=w2336:string)
                                n1843 = Decimal String To Number(string=w2336) -> (number=w2335:i32)  [unwired: 2 in, 1 out]
                                n1844 = In Range and Coerce(upper limit="DEC Max", x=w2335, lower limit="DEC Min") -> (In Range?=w2333:bool)  [unwired: 1 out]
                                n1845 = case shown="True" w2333 {
                                tunnel: w2334 -> [w2340 w2343]
                                tunnel: [w2340 w2342] -> w2332
                                tunnel: w2331 -> [_ w2341]
                                frame False {
                                }
                                frame True {
                                n1846 = Build Array (concatenate)(w2343, w2341) -> (w2342:string[][])
                                }
                                }
                              }
                            }
                            frame #2 {
                              # "Filtro de MAG"
                              n1847 = Index Array(array=w2344, index (col)=3 ("disabled index (col)")) -> (element=w2347:string[])  [unwired: 1 in]
                              n1848 = for {
                                tunnel: w2347 -> [w2349] mode=indexing
                                shift-right: [w2353] -> w2345
                                shift-left: string[][] [] ("Item Names") -> [w2357]
                                tunnel: w2344 -> [w2355] mode=indexing
                                n1849 = Fract/Exp String To Number(use system decimal point (T)=FALSE, string=w2349) -> (number=w2352:dbl)  [unwired: 2 in, 1 out]
                                n1850 = In Range and Coerce(upper limit="MAG Max", x=w2352, lower limit="MAG Min") -> (In Range?=w2356:bool)  [unwired: 1 out]
                                n1851 = case shown="True" w2356 {
                                tunnel: w2357 -> [w2358 w2361]
                                tunnel: [w2358 w2360] -> w2353
                                tunnel: w2355 -> [_ w2359]
                                frame False {
                                }
                                frame True {
                                n1852 = Build Array (concatenate)(w2361, w2359) -> (w2360:string[][])
                                }
                                }
                              }
                            }
                            frame #3 {
                              w2362 = 0 ("index")
                              n1853 = local write "subarray"(w2370) -> ()
                              n1854 = Array Size(array=w2370) -> (size(s)=w2382:i32[])
                              n1855 = Index Array(array=w2382, index=0) -> (element=w2375:i32)
                              n1856 = local write "Tot Linhas"(w2375) -> ()
                              n1857 = local write "Slide old"(w2362) -> ()
                              n1858 = local write "Slide"(w2362) -> ()
                              n1859 = Array Subset(array=w2370, index (row)=w2362, length (row)=11 ("length"), index (col)=0 ("index"), length (col)=8 ("index")) -> (w2371:string[][])
                              n1860 = property on="Multicolumn Listbox" class="MCListbox (strict)"("Item Names"=w2371) -> ()  [unwired: 2 in, 2 out]
                              n1861 = Quotient & Remainder(x=10000, y=w2375) -> (floor(x/y)=w2379:i32)  [unwired: 1 out]
                              n1862 = Divide(x=w2379, y=1000) -> (x/y=w2377:dbl)
                              n1863 = control-ref of="Erro"() -> (w2366:refnum<vi>)
                              n1864 = Multiply(x=w2377, y=24.0) -> (x*y=w2364:dbl)
                              n1865 = property class="Bool (strict)"(reference=w2366, "Boolean Text.Text"="") -> ()  [unwired: 1 in, 2 out]
                              n1866 = Decrement(x=w2364) -> (x-1=w2363:dbl)
                              n1867 = property on="Slide" class="Slide (strict)"("Data Entry Limits:Increment"=w2363) -> ()  [unwired: 2 in, 2 out]
                              n1868 = local write "Erro"(FALSE ("Erro")) -> ()
                            }
                          }
                        }
                        frame "erro", Default {
                          n1869 = control-ref of="Erro"() -> (w2384:refnum<vi>)
                          n1870 = property class="Bool (strict)"(reference=w2384, "Boolean Text.Text"="ERROR") -> ()  [unwired: 1 in, 2 out]
                          n1871 = local write "Erro"(TRUE ("Erro")) -> ()
                        }
                        frame "fim" {
                          n1872 = local read "RA Max 2"() -> (w2389:i32)
                          n1873 = local read "RA Min 2"() -> (w2388:i32)
                          n1874 = Number To Decimal String(number=w2388) -> (decimal integer string=w2391:string)  [unwired: 1 in]
                          n1875 = Number To Decimal String(number=w2389) -> (decimal integer string=w2390:string)  [unwired: 1 in]
                          n1876 = local write "ScaleMin"(w2391) -> ()
                          n1877 = local write "ScaleMax"(w2390) -> ()
                        }
                      }
                    }
                  }
                }
              }
            }
          }
          frame " INSTRUMENT " {
            n1878 = case shown="\"Coude\", Default" "TabInstrumento" {
              frame "Casseg." {
                w2405 = u16 13 items=["Alarme", "Atencao", "Erro", "Ocupado", "PosSecund", "PosConj#3", "MovFoco", "MovCjto#3", "Mov#4", "Mov#3", "Mov#2", "EspLamp", "HE", "NE", "EspLampRepouso", "EspLampCalibra"] ("NomeStatus")
                w2404 = u16 12 items=["Alarme", "Atencao", "Erro", "Ocupado", "PosSecund", "PosConj#3", "MovFoco", "MovCjto#3", "Mov#4", "Mov#3", "Mov#2", "EspLamp", "HE", "NE", "EspLampRepouso", "EspLampCalibra"] ("NomeStatus")
                w2406 = u16 15 items=["Alarme", "Atencao", "Erro", "Ocupado", "PosSecund", "PosConj#3", "MovFoco", "MovCjto#3", "Mov#4", "Mov#3", "Mov#2", "EspLamp", "HE", "NE", "EspLampRepouso", "EspLampCalibra"] ("NomeStatus")
                w2407 = u16 14 items=["Alarme", "Atencao", "Erro", "Ocupado", "PosSecund", "PosConj#3", "MovFoco", "MovCjto#3", "Mov#4", "Mov#3", "Mov#2", "EspLamp", "HE", "NE", "EspLampRepouso", "EspLampCalibra"] ("NomeStatus")
                w2408 = u16 11 items=["Alarme", "Atencao", "Erro", "Ocupado", "PosSecund", "PosConj#3", "MovFoco", "MovCjto#3", "Mov#4", "Mov#3", "Mov#2", "EspLamp", "HE", "NE", "EspLampRepouso", "EspLampCalibra"] ("NomeStatus")
                # "Cassegrain"
                n1879 = event shown="[3] \"Sent_EspLampCass\": Value Change" {
                  selector: _ -> [_ _ _ _]
                  dyn-events: _ -> [_ _ _ _]
                  timeout: 10 -> [_ _ _ _]
                  event Timeout {
                    n1880 = event-data() -> ()  [unwired: 1 in, 2 out]
                  }
                  event "Ne": Value Change {
                    w2435 = u16 3 items=["ZERO", "AH", "DEC", "TUBO", "CUP"] ("Controlador")
                    n1881 = event-data() -> ()  [unwired: 1 in, 1 out]
                    n1882 = case shown="True" "Ne" {
                      tunnel: ["LAMP_NE" "LAMP_NE"] -> w2434
                      tunnel: ["DESLIGAR" "LIGAR"] -> w2433
                      frame False {
                      }
                      frame True {
                      }
                    }
                    n1883 = call "Monta Comando.vi"("Comando"=w2433, "Dispositivo"=w2434, "Controlador"=w2435) -> ()  [unwired: 4 in, 3 out]
                  }
                  event "He-Ar": Value Change {
                    w2443 = u16 3 items=["ZERO", "AH", "DEC", "TUBO", "CUP"] ("Controlador")
                    n1884 = event-data() -> ()  [unwired: 1 in, 1 out]
                    n1885 = case shown="False" "He-Ar" {
                      tunnel: ["LAMP_HE" "LAMP_HE"] -> w2442
                      tunnel: ["DESLIGAR" "LIGAR"] -> w2441
                      frame False {
                      }
                      frame True {
                      }
                    }
                    n1886 = call "Monta Comando.vi"("Comando"=w2441, "Dispositivo"=w2442, "Controlador"=w2443) -> ()  [unwired: 4 in, 3 out]
                  }
                  event "Sent_EspLampCass": Value Change {
                    w2451 = u16 3 items=["ZERO", "AH", "DEC", "TUBO", "CUP"] ("Controlador")
                    n1887 = event-data() -> ()  [unwired: 1 in, 1 out]
                    n1888 = property on="SlideEcass" class="Slide (strict)"("Visible"=TRUE) -> ()  [unwired: 2 in, 2 out]
                    n1889 = case shown="False" "Sent_EspLampCass" {
                      tunnel: ["ESP_LAMP" "ESP_LAMP"] -> w2450
                      tunnel: ["RECUAR" "AVANCAR"] -> w2449
                      frame False {
                      }
                      frame True {
                      }
                    }
                    n1890 = property on="stopEcass" class="Bool"("Visible"=FALSE) -> ()  [unwired: 2 in, 2 out]
                    n1891 = call "Monta Comando.vi"("Comando"=w2449, "Dispositivo"=w2450, "Controlador"=w2451) -> ()  [unwired: 4 in, 3 out]
                    "SlideEcass" <- u8 8 ("Slide")
                  }
                }
                n1892 = call "Bit Status TUBO.vi"("NomeStatus"=w2404) -> ("StatBit"=→"LedHe":bool)
                n1893 = call "Bit Status TUBO.vi"("NomeStatus"=w2405) -> ("StatBit"=→"LedNe":bool)
                n1894 = call "Bit Status TUBO.vi"("NomeStatus"=w2408) -> ("StatBit"=w2403:bool)
                n1895 = call "Bit Status TUBO.vi"("NomeStatus"=w2407) -> ("StatBit"=w2402:bool)
                n1896 = call "Bit Status TUBO.vi"("NomeStatus"=w2406) -> ("StatBit"=w2401:bool)
                n1897 = And(x=w2403, y=w2402) -> (x .and. y?=w2400:bool)
                "LedRep" <- w2400
                n1898 = And(x=w2403, y=w2401) -> (x .and. y?=w2399:bool)
                "LedCal" <- w2399
                n1899 = property on="SlideEcass" class="Slide (strict)"() -> ("Visible"=w2398:bool)  [unwired: 2 in, 2 out]
                n1900 = Or(x=w2400, y=w2399) -> (x .or. y?=w2410:bool)
                n1901 = Or(x=w2402, y=w2401) -> (x .or. y?=w2413:bool)
                n1902 = Not(x=w2403) -> (.not. x?=w2412:bool)
                n1903 = And(x=w2398, y=w2410) -> (x .and. y?=w2409:bool)
                n1904 = And(x=w2412, y=w2413) -> (x .and. y?=w2411:bool)
                n1905 = case shown="True" "stopEcass" {
                  frame False {
                  }
                  frame True {
                    w2430 = FALSE
                    w2429 = u8 0 ("Disabled")
                    w2428 = u16 3 items=["ZERO", "AH", "DEC", "TUBO", "CUP"] ("Controlador")
                    n1906 = call "Monta Comando.vi"("Comando"="DESLIGAR", "Dispositivo"="ESP_LAMP", "Controlador"=w2428) -> ()  [unwired: 4 in, 3 out]
                    n1907 = property on="Sent_EspLampCass" class="Bool (strict)"("Disabled"=w2429) -> ()  [unwired: 2 in, 2 out]
                    n1908 = property on="Ne" class="Bool (strict)"("Disabled"=w2429) -> ()  [unwired: 2 in, 2 out]
                    n1909 = property on="He-Ar" class="Bool (strict)"("Disabled"=w2429) -> ()  [unwired: 2 in, 2 out]
                    n1910 = property on="SlideEcass" class="Slide (strict)"("Visible"=w2430) -> ()  [unwired: 2 in, 2 out]
                    n1911 = property on="stopEcass" class="Bool"("Visible"=w2430) -> ()  [unwired: 2 in, 2 out]
                  }
                }
                n1912 = case shown="True" w2409 {
                  frame False {
                  }
                  frame True {
                    w2431 = u8 0 ("Disabled")
                    n1913 = property on="Sent_EspLampCass" class="Bool (strict)"("Disabled"=w2431) -> ()  [unwired: 2 in, 2 out]
                    n1914 = property on="He-Ar" class="Bool (strict)"("Disabled"=w2431) -> ()  [unwired: 2 in, 2 out]
                    n1915 = property on="Ne" class="Bool (strict)"("Disabled"=w2431) -> ()  [unwired: 2 in, 2 out]
                    n1916 = property on="SlideEcass" class="Slide (strict)"("Visible"=FALSE) -> ()  [unwired: 2 in, 2 out]
                  }
                }
                n1917 = case shown="True" w2411 {
                  frame False {
                  }
                  frame True {
                    w2415 = u8 2 ("Disabled")
                    n1918 = local read "SlideEcass"() -> (w2416:u8)
